vi "DAQmx.Create AI Tasks.vi"(8 "error in":errorcluster, 11 "DAQmx in":refnum<class "DAQmx.lvclass">) -> (0 "error out":errorcluster, 3 "DAQmx out":refnum<class "DAQmx.lvclass">)   [LabVIEW 2019, in "DAQmx.lvclass"]
uses:
  DAQmx.lvclass
  typedefs/DAQ.Config.AI--Cluster--Array.ctl
  typedefs/DAQ.Config.AI--Cluster.ctl
  typedefs/DAQ.Config.AI.Coupling--enum.ctl
  typedefs/DAQ.Config.AI.Range--enum.ctl
  typedefs/DAQ.Config.Device Type--enum.ctl
  DAQmx.lvclass/DAQmx.ctl
  <vilib>/DAQmx/create/channels.llb/DAQmx Create Channel (AI-Voltage-Basic).vi
  <resource>/objmgr/daqmx.rc
panel:
  out "AI":T1 {"input terminal configuration" items=[""=-1, "Differential"=10106, "Pseudodifferential"=12529]; "Coupling" items=[""=0, "AC"=10045, "DC"=10050, "GND"=10066]}
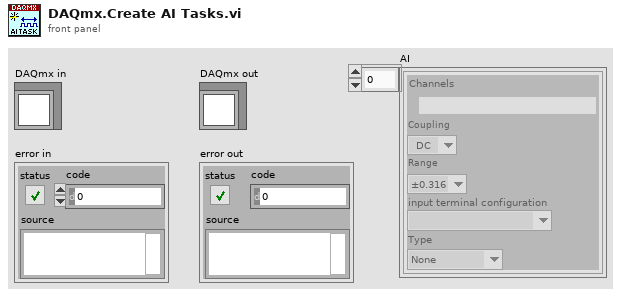
[diagram p1: front panel]
types:
  T1 = typedef "DAQmx.lvclass/DAQ.Config.AI--Cluster--Array.ctl" = T2[]
  T2 = typedef "DAQmx.lvclass/DAQ.Config.AI--Cluster.ctl" = cluster{"Channels":tag, "Coupling":T3, "Range":T4, "input terminal configuration":i32, "Type":T5}
  T3 = typedef "DAQmx.lvclass/DAQ.Config.AI.Coupling--enum.ctl" = u16
  T4 = typedef "DAQmx.lvclass/DAQ.Config.AI.Range--enum.ctl" = enum16{"±0.316", "±1.00", "±3.16", "±10.0", "±31.6", "±42.4", ""}
  T5 = typedef "DAQmx.lvclass/DAQ.Config.Device Type--enum.ctl" = enum16{"None", "USB-4431", "PXI-446x"}
  T6 = typedef "DAQmx.lvclass/DAQmx.Channel Map--Cluster.ctl" = cluster{"task":refnum<k21>, "Device":tag, "Offset":u32, "Count":u32}
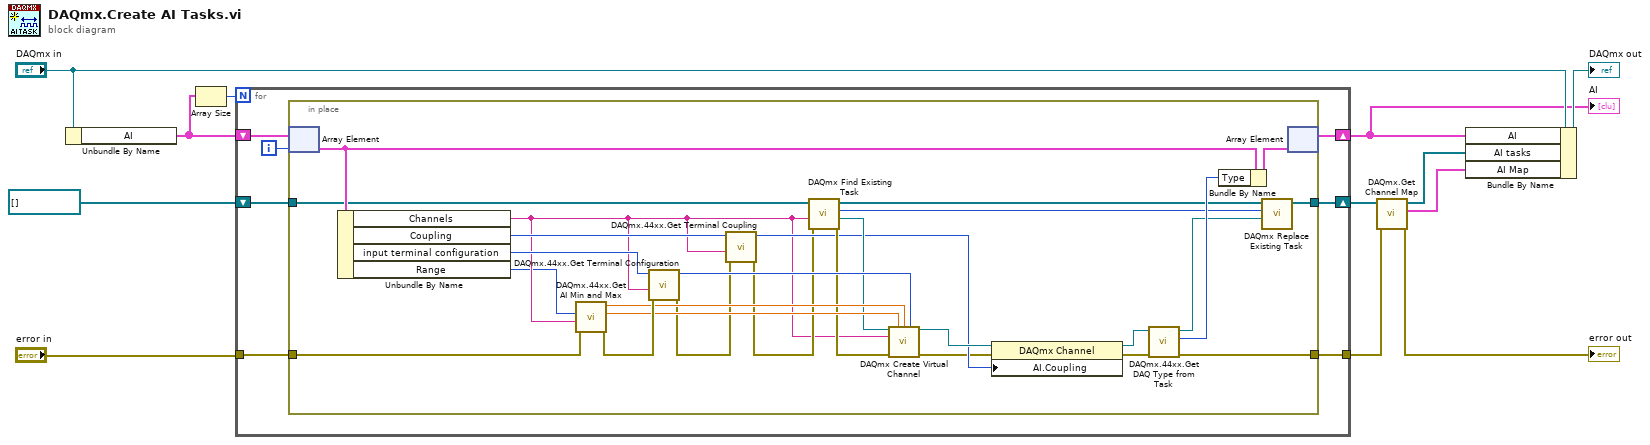
[diagram p0: block diagram]
diagram:
  n1 = Unbundle By Name("DAQmx in") -> ("AI"=w7:T1)
  n2 = Array Size(array=w7) -> (size(s)=w8:i32)
  n3 = for {
    N: w8 -> [_]
    tunnel: "error in" -> [w19]
    tunnel: [w16] -> w5
    shift-right: [w18] -> w2
    shift-left: refnum<k21>[] [] -> [w17]
    shift-right: [w13] -> w6
    shift-left: w7 -> [w15]
    i -> [w14]
    n4 = in-place {
      in-place-border: w19 -> [w46]
      in-place-border: [w44] -> w18
      in-place-border: w17 -> [w37]
      in-place-border: [w41] -> w16
      n5 = in-place-array #1(w15, w14) -> (w39:T2)
      n6 = Unbundle By Name(w39) -> ("Channels"=w21:tag, "Coupling"=w26:T3, "input terminal configuration"=w31:i32, "Range"=w20:T4)
      n7 = call "DAQmx.44xx.Get AI Min and Max.vi"("error in (no error)"=w46, "AI.channels"=w21, "AI.Range"=w20) -> ("error out"=w34:errorcluster, "AI.Max"=w33:dbl, "AI.Min"=w32:dbl)  [unwired: 6 in]
      n8 = call "DAQmx.44xx.Get Terminal Configuration.vi"("error in (no error)"=w34, "Channel in"=w21, "terminal configuration in"=w31) -> ("error out"=w23:errorcluster, "terminal configuration out"=w35:i32)  [unwired: 7 in]
      n9 = call "DAQmx.44xx.Get Terminal Coupling.vi"("error in (no error)"=w23, "Channel in"=w21, "Coupling in"=w26) -> ("error out"=w22:errorcluster, "AI.Coupling"=w25:i32)  [unwired: 7 in]
      n10 = call "DAQmx Find Existing Task.vi"("error in (no error)"=w22, "Channels"=w21, "Tasks in"=w37) -> ("error out"=w27:errorcluster, "Task out"=w28:refnum<k21>, "Task Index"=w30:i32, "Tasks out"=w29:refnum<k21>[])  [unwired: 5 in]
      n11 = call-poly <vilib>:"DAQmx Create Virtual Channel.vi"("task in"=w28, "maximum value"=w33, "minimum value"=w32, "input terminal configuration"=w35, "physical channels"=w21, "error in"=w27) -> ("task out"=w36:refnum<k21>, "error out"=w24:errorcluster)  [unwired: 8 in]
      n12 = property class="DAQmx Channel"(reference=w36, error in=w24, "AI.Coupling"=w25) -> (reference out=w40:refnum<k21>, error out=w43:errorcluster)
      n13 = call "DAQmx.44xx.Get DAQ Type from Task.vi"("error in (no error)"=w43, "Task in"=w40) -> ("error out"=w41:errorcluster, "DAQ Type"=w45:T5, "Task out"=w42:refnum<k21>)  [unwired: 5 in, 2 out]
      n14 = Bundle By Name(cluster=w39, "Type"=w45) -> (w38:T2)
      n15 = call "DAQmx Replace Existing Task.vi"("Task in"=w42, "Task Index"=w30, "Tasks in"=w29) -> ("Tasks out"=w44:refnum<k21>[])  [unwired: 8 in]
      n16 = in-place-array #1(w38) -> (w13:T1)  [unwired: 1 out]
    }
  }
  "AI" <- w6
  n17 = call "DAQmx.Get Channel Map.vi"("error in (no error)"=w5, "tasks in"=w2) -> ("error out"=→"error out":errorcluster, "Channel Map"=w3:T6[], "tasks out"=w1:refnum<k21>[])  [unwired: 7 in]
  n18 = Bundle By Name(cluster="DAQmx in", "AI"=w6, "AI tasks"=w1, "AI Map"=w3) -> (→"DAQmx out":refnum<class "DAQmx.lvclass">)
